vi "Final.vi"(0 "laser1":i32, 1 "laser2":i32, 2 "User1_float":dbl, 3 "Mode":i32, 4 "laser3":i32, 5 "laser4":i32, 6 "User2_int":i32, 7 "k":i32=1, 8 "If Scanning":dbl format="%#_13g", 9 "DC Offset X":dbl=5.0 format="%#_13g", 10 "ExposureTime(ms)":dbl, 12 "TriggerDelay(ms)":dbl=100.0, 13 "LoopDelay(second)":dbl, 14 "DC Offset Y":dbl=5.0 format="%#_13g", 15 "VoltageScanningChannel":tag="Dev2/ao0:3", 16 "LaserTriggerChannel":tag="Dev2/port0", 17 "frequency":dbl=30.0 caption="Frequency" format="%.6f", 18 "VXPX":dbl=0.08805 format="%#_13g", 19 "VYPY":dbl=0.10448 format="%#_13g", 20 "z_num":dbl format="%#_13g", 21 "delta_z(x1um)":dbl format="%#_13g", 22 "XShiftRatio":dbl=-0.01 format="%#_13g", 23 "YShiftRatio":dbl=0.01258 format="%#_13g", 24 "停止":bool, 25 "RotationAlpha":dbl=23.3, 27 "RotationBeta":dbl=113.3) -> ()   [LabVIEW 2019]
uses:
  <vilib>/DAQmx/write.llb/DAQmx Write (Digital 1D U32 1Chan NSamp).vi
  <vilib>/DAQmx/write.llb/DAQmx Write (Analog 2D DBL NChan NSamp).vi
  <vilib>/DAQmx/create/channels.llb/DAQmx Create Channel (AO-Voltage-Basic).vi
  <vilib>/DAQmx/create/channels.llb/DAQmx Create Channel (DO-Digital Output).vi
  <vilib>/DAQmx/configure/timing.llb/DAQmx Timing (Sample Clock).vi
  <vilib>/DAQmx/miscellaneous.llb/DAQmx Fill In Error Info.vi
  <vilib>/DAQmx/create/channels.llb/DAQmx Create Channel (CO-Pulse Generation-Frequency).vi
  <vilib>/DAQmx/configure/timing.llb/DAQmx Timing (Implicit).vi
  Global 6.vi
panel:
  out "Laser_status":i32[](array[numeric])
  out "Camera_trigger":i32[](array[numeric])
  out "XY Graph":cluster{"Y":dbl[], "Y":dbl[]}[](graph) caption="XY图"
  out "Scanning_index":dbl[][](array[numeric])=[[0.005349794238683128, 0.005349794238683128, 0.005349794238683128, 0.005349794238683128, -0.0, -0.0, -0.0, -0.0, -0.005349794238683128, -0.005349794238683128, -0.005349794238683128, -0.005349794238683128, -0.005349794238683128, -0.005349794238683128, -0.005349794238683128, -0.005349794238683128, -0.005349794238683128, -0.005349794238683128, -0.005349794238683128, -0.005349794238683128, -0.0, -0.0, -0.0, -0.0, 0.005349794238683128, 0.005349794238683128, 0.005349794238683128, 0.005349794238683128, 0.005349794238683128, 0.005349794238683128, 0.005349794238683128, 0.005349794238683128, -0.0, -0.0, -0.0, -0.0], [0.0020833333333333333, 0.0020833333333333333, 0.0020833333333333333, 0.0020833333333333333, 0.0020833333333333333, 0.0020833333333333333, 0.0020833333333333333, 0.0020833333333333333, 0.0020833333333333333, 0.0020833333333333333, 0.0020833333333333333, 0.0020833333333333333, -0.0, -0.0, -0.0, -0.0, -0.0020833333333333333, -0.0020833333333333333, -0.0020833333333333333, -0.0020833333333333333, -0.0020833333333333333, -0.0020833333333333333, -0.0020833333333333333, -0.0020833333333333333, -0.0020833333333333333, -0.0020833333333333333, -0.0020833333333333333, -0.0020833333333333333, -0.0, -0.0, -0.0, -0.0, -0.0, -0.0, -0.0, -0.0]]
  out "Scanning_voltage":dbl[][](array[numeric])=[[0.005349794238683128, 0.005349794238683128, 0.005349794238683128, 0.005349794238683128, -0.0, -0.0, -0.0, -0.0, -0.005349794238683128, -0.005349794238683128, -0.005349794238683128, -0.005349794238683128, -0.005349794238683128, -0.005349794238683128, -0.005349794238683128, -0.005349794238683128, -0.005349794238683128, -0.005349794238683128, -0.005349794238683128, -0.005349794238683128, -0.0, -0.0, -0.0, -0.0, 0.005349794238683128, 0.005349794238683128, 0.005349794238683128, 0.005349794238683128, 0.005349794238683128, 0.005349794238683128, 0.005349794238683128, 0.005349794238683128, -0.0, -0.0, -0.0, -0.0], [0.0020833333333333333, 0.0020833333333333333, 0.0020833333333333333, 0.0020833333333333333, 0.0020833333333333333, 0.0020833333333333333, 0.0020833333333333333, 0.0020833333333333333, 0.0020833333333333333, 0.0020833333333333333, 0.0020833333333333333, 0.0020833333333333333, -0.0, -0.0, -0.0, -0.0, -0.0020833333333333333, -0.0020833333333333333, -0.0020833333333333333, -0.0020833333333333333, -0.0020833333333333333, -0.0020833333333333333, -0.0020833333333333333, -0.0020833333333333333, -0.0020833333333333333, -0.0020833333333333333, -0.0020833333333333333, -0.0020833333333333333, -0.0, -0.0, -0.0, -0.0, -0.0, -0.0, -0.0, -0.0]]
  out "z_voltage":dbl[](array[numeric])
  out "Scanning_voltage_correct":dbl[][](array[numeric])=[[0.005349794238683128, 0.005349794238683128, 0.005349794238683128, 0.005349794238683128, -0.0, -0.0, -0.0, -0.0, -0.005349794238683128, -0.005349794238683128, -0.005349794238683128, -0.005349794238683128, -0.005349794238683128, -0.005349794238683128, -0.005349794238683128, -0.005349794238683128, -0.005349794238683128, -0.005349794238683128, -0.005349794238683128, -0.005349794238683128, -0.0, -0.0, -0.0, -0.0, 0.005349794238683128, 0.005349794238683128, 0.005349794238683128, 0.005349794238683128, 0.005349794238683128, 0.005349794238683128, 0.005349794238683128, 0.005349794238683128, -0.0, -0.0, -0.0, -0.0], [0.0020833333333333333, 0.0020833333333333333, 0.0020833333333333333, 0.0020833333333333333, 0.0020833333333333333, 0.0020833333333333333, 0.0020833333333333333, 0.0020833333333333333, 0.0020833333333333333, 0.0020833333333333333, 0.0020833333333333333, 0.0020833333333333333, -0.0, -0.0, -0.0, -0.0, -0.0020833333333333333, -0.0020833333333333333, -0.0020833333333333333, -0.0020833333333333333, -0.0020833333333333333, -0.0020833333333333333, -0.0020833333333333333, -0.0020833333333333333, -0.0020833333333333333, -0.0020833333333333333, -0.0020833333333333333, -0.0020833333333333333, -0.0, -0.0, -0.0, -0.0, -0.0, -0.0, -0.0, -0.0]]
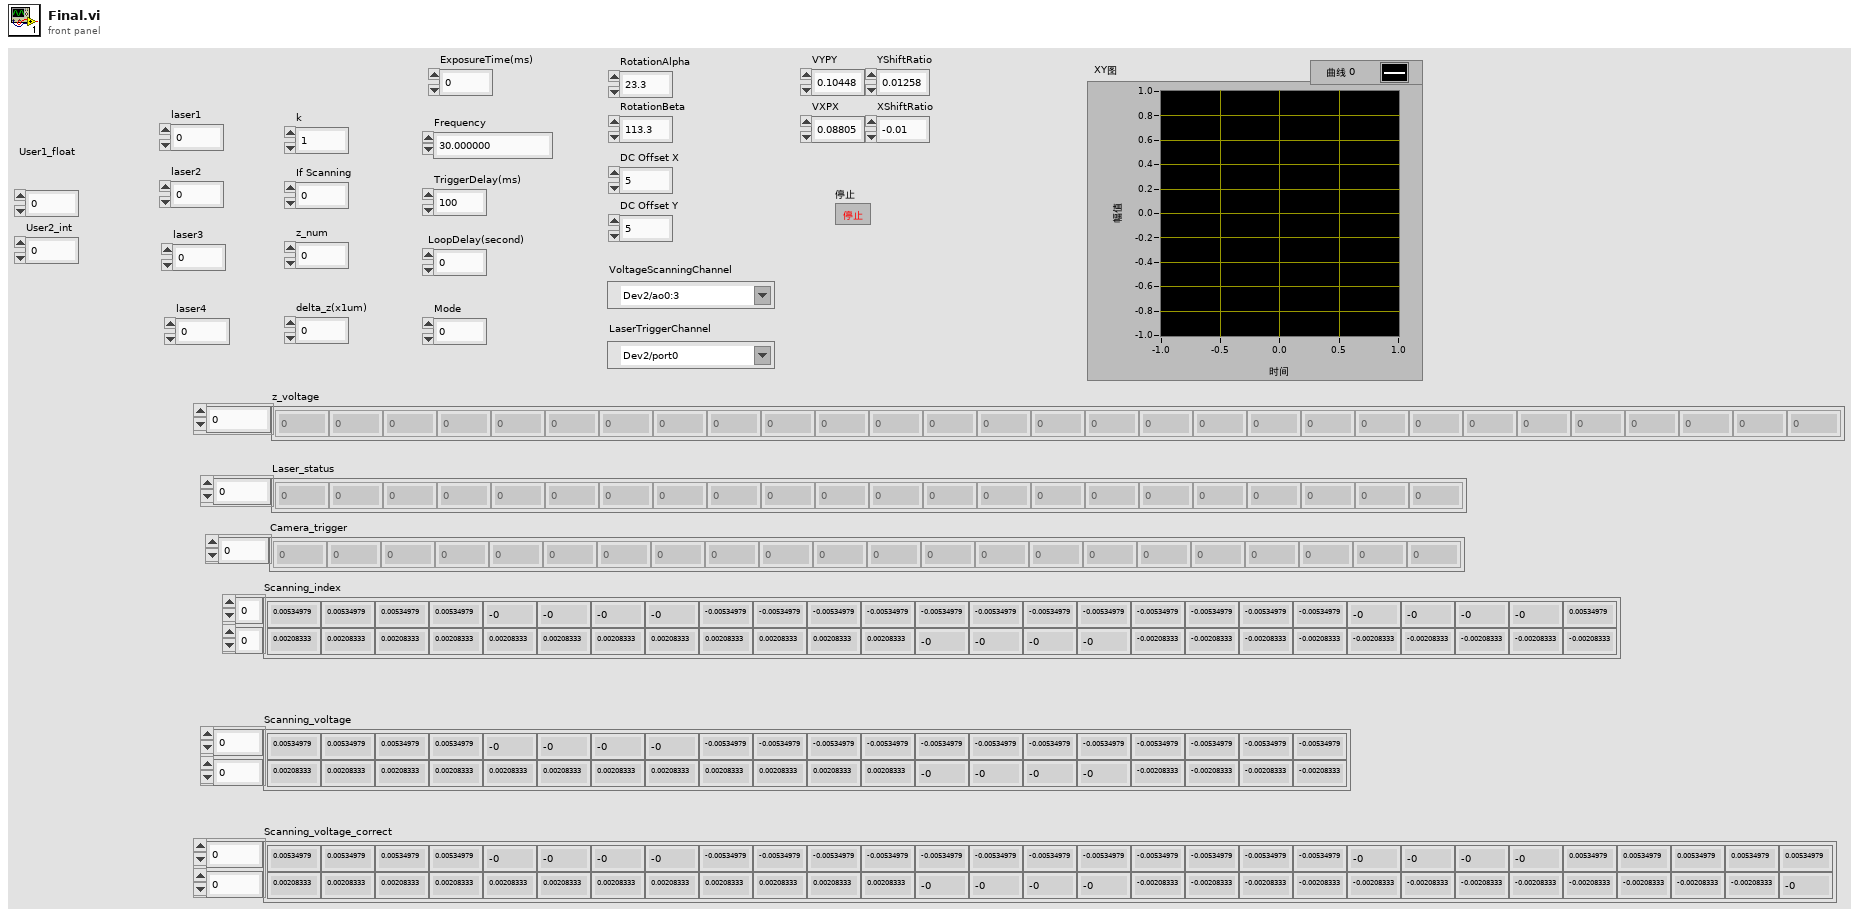
[diagram p1: front panel]
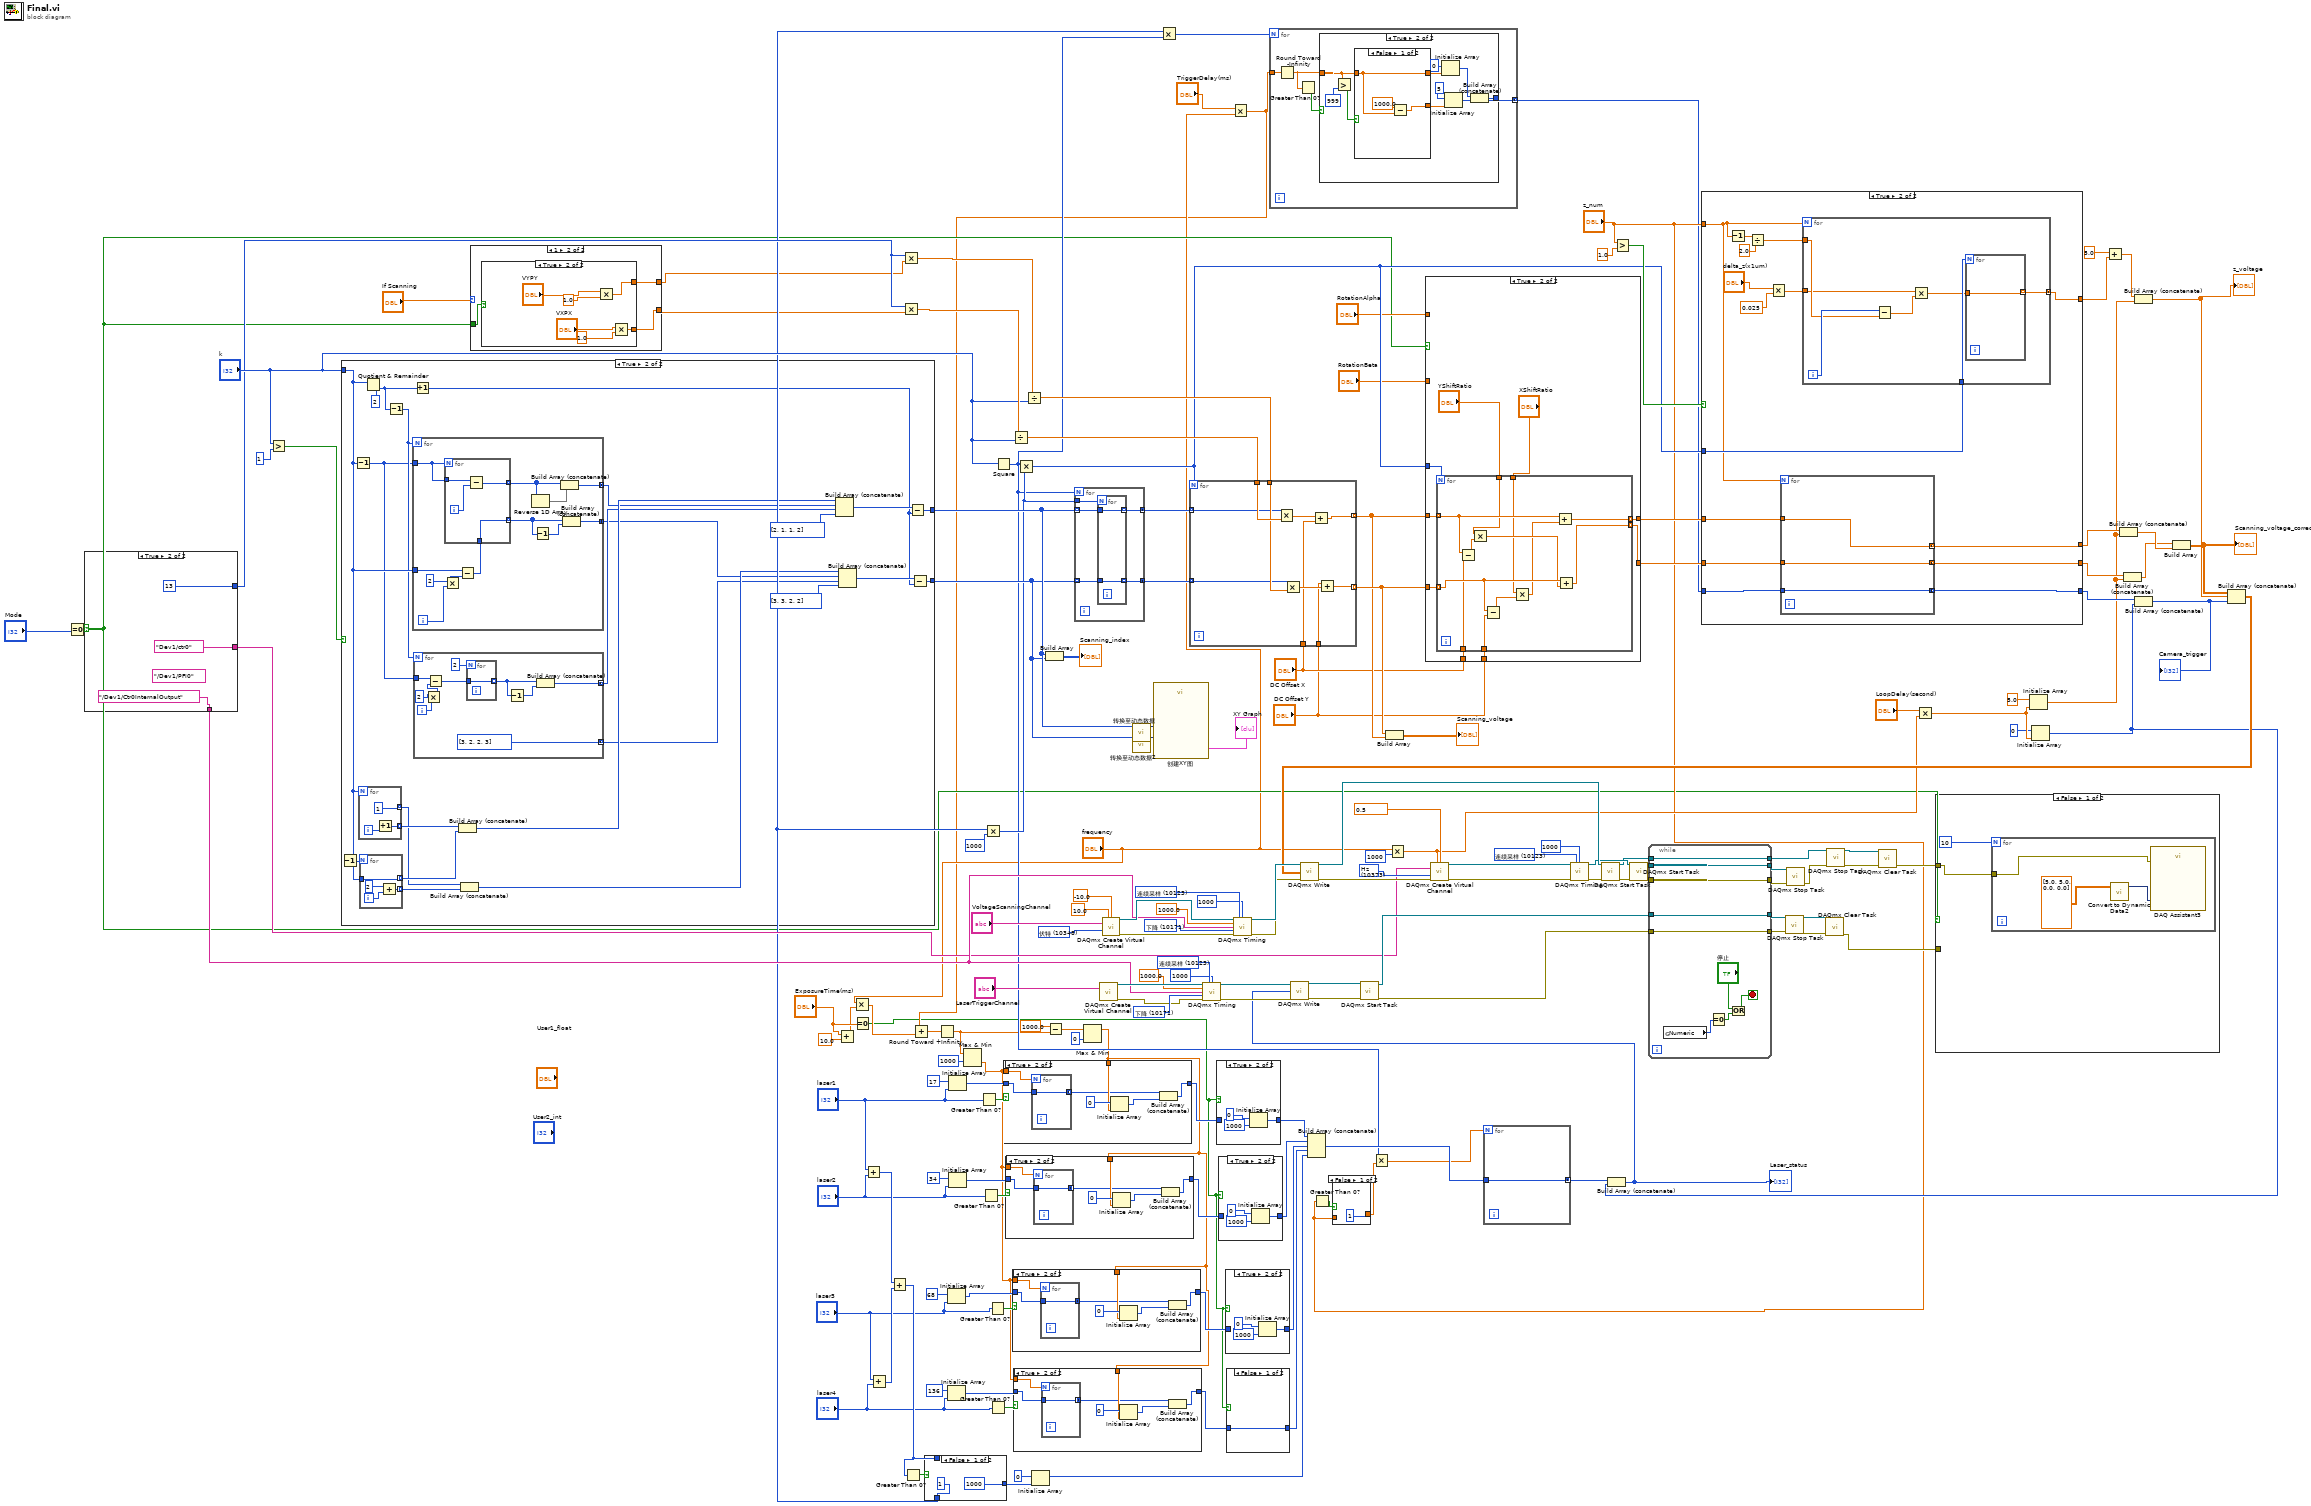
[diagram p0: block diagram]
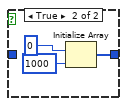
[diagram p2: hidden frame]
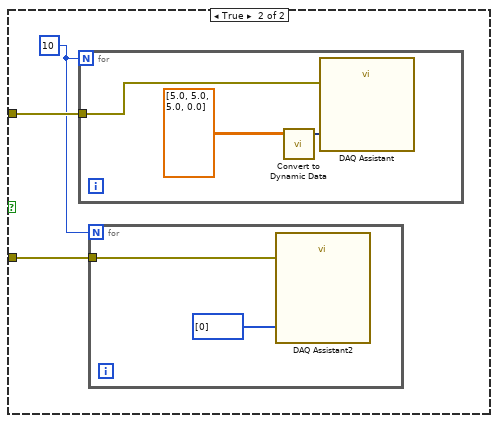
[diagram p10: hidden frame]
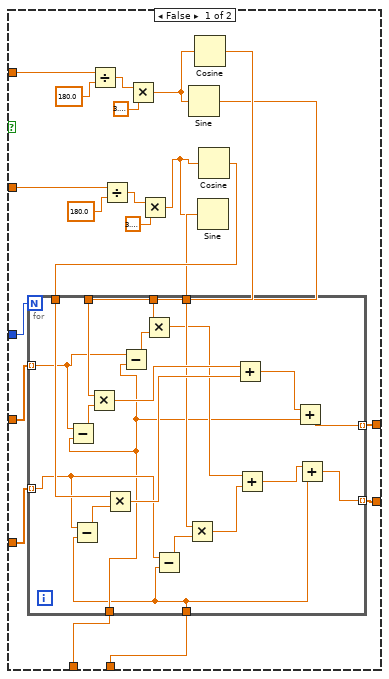
[diagram p11: hidden frame]
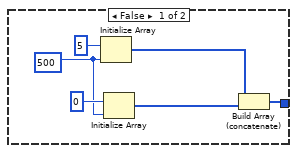
[diagram p12: hidden frame]
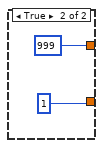
[diagram p13: hidden frame]
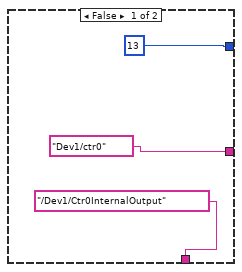
[diagram p14: hidden frame]
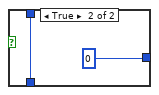
[diagram p16: hidden frame]
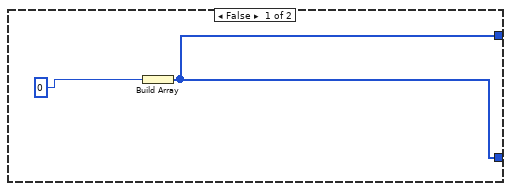
[diagram p17: hidden frame]
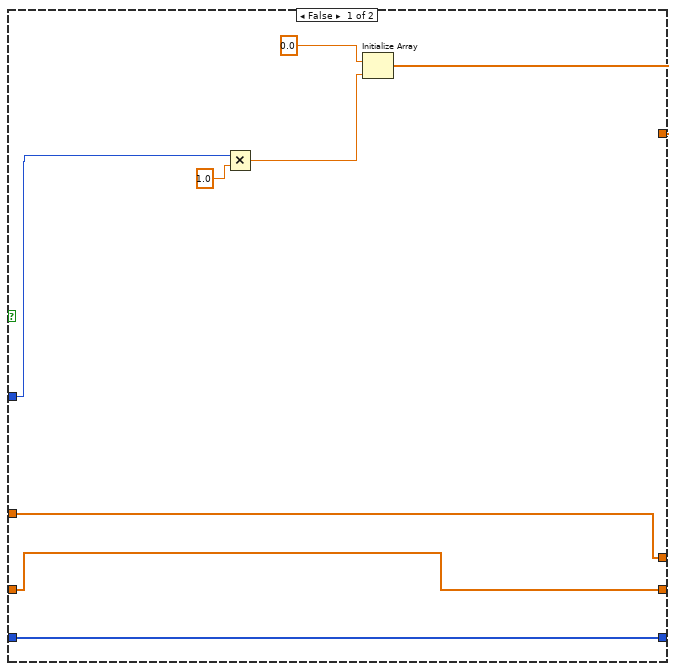
[diagram p18: hidden frame]
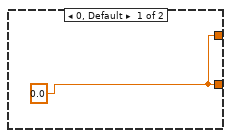
[diagram p19: hidden frame]
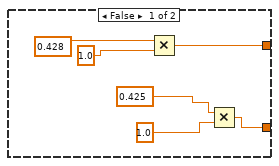
[diagram p20: hidden frame]
diagram:
  w134 = 10171 items=["上升"=10280, "下降"=10171] ("active edge")
  w136 = 10123 items=["有限采样"=10178, "连续采样"=10123, "硬件定时单点"=12522] ("sample mode")
  w148 = 10123 items=["有限采样"=10178, "连续采样"=10123, "硬件定时单点"=12522] ("sample mode")
  w159 = 10373 items=["Hz"=10373] ("units")
  w161 = 10348 items=["伏特"=10348, "来自自定义换算"=10065] ("units")
  w164 = 10171 items=["上升"=10280, "下降"=10171] ("active edge")
  w166 = 10123 items=["有限采样"=10178, "连续采样"=10123, "硬件定时单点"=12522] ("sample mode")
  n1 = Equal To 0?(x="Mode") -> (x = 0?=w40:bool)
  n2 = case shown="True" w40 {
    tunnel: [13 13] -> w55
    tunnel: [tag "/Dev1/Ctr0InternalOutput" ("source") tag "/Dev1/Ctr0InternalOutput" ("source")] -> w54
    tunnel: [tag "Dev1/ctr0" ("counter") tag "Dev1/ctr0" ("counter")] -> w52
    frame False {
    }
    frame True {
      (unwired) tag "/Dev1/PFI0" ("source")
    }
  }
  n3 = Greater?(x="k", y=1) -> (0:w95:bool)
  n4 = case shown="True" w95 {
    tunnel: "k" -> [_ w191]
    tunnel: [w173 w176] -> w101
    tunnel: [w173 w175] -> w99
    frame False {
      n5 = Build Array(0) -> (w173:i32[])
    }
    frame True {
      n6 = Decrement(x=w191) -> (x-1=w196:i32)
      n7 = Decrement(x=w191) -> (x-1=w189:i32)
      n8 = for {
        N: w191 -> [_]
        tunnel: [1] -> w193 mode=indexing
        tunnel: [w229] -> w195 mode=indexing
        i -> [w230]
        n9 = Increment(x=w230) -> (x+1=w229:i32)
      }
      n10 = for {
        N: w196 -> [_]
        tunnel: [w228] -> w194 mode=indexing
        tunnel: w191 -> [w228]
        tunnel: [w225] -> w192 mode=indexing
        i -> [w227]
        n11 = Add(x=2, y=w227) -> (x+y=w225:i32)
      }
      n12 = Quotient & Remainder(x=w191, y=2) -> (floor(x/y)=w180:i32)  [unwired: 1 out]
      n13 = Decrement(x=w180) -> (x-1=w190:i32)
      n14 = for {
        N: w190 -> [_]
        tunnel: w189 -> [w220]
        tunnel: [w217] -> w187 mode=concatenating
        tunnel: w191 -> [w215]
        tunnel: [w209] -> w182 mode=concatenating
        i -> [w213]
        n15 = Multiply(x=2, y=w213) -> (x*y=w216:i32)
        n16 = Subtract(x=w215, y=w216) -> (x-y=w212:i32)
        n17 = for {
          N: w220 -> [_]
          tunnel: w220 -> [w224]
          tunnel: [w223] -> w218 mode=indexing
          tunnel: w212 -> [w221]
          tunnel: [w221] -> w211 mode=indexing
          i -> [w222]
          n18 = Subtract(x=w224, y=w222) -> (x-y=w223:i32)
        }
        n19 = Reverse 1D Array(array=w218) -> (reversed array=w219:i32[])
        n20 = Decrement(x=w211) -> (x-1=w210:i32[])
        n21 = Build Array (concatenate)(w218, w219) -> (w217:i32[])
        n22 = Build Array (concatenate)(w211, w210) -> (w209:i32[])
      }
      n23 = Increment(x=w180) -> (x+1=w177:i32)
      n24 = for {
        N: w190 -> [_]
        tunnel: w189 -> [w206]
        tunnel: [w202] -> w186 mode=concatenating
        tunnel: [i32[] [3, 2, 2, 3]] -> w181 mode=concatenating
        i -> [w200]
        n25 = Multiply(x=2, y=w200) -> (x*y=w198:i32)
        n26 = Subtract(x=w206, y=w198) -> (x-y=w205:i32)
        n27 = for {
          N: 2 -> [_]
          tunnel: [w208] -> w203 mode=indexing
          tunnel: w205 -> [w208]
        }
        n28 = Decrement(x=w203) -> (x-1=w204:i32[])
        n29 = Build Array (concatenate)(w203, w204) -> (w202:i32[])
      }
      n30 = Build Array (concatenate)(w195, w194) -> (w188:i32[])
      n31 = Build Array (concatenate)(w193, w192) -> (w183:i32[])
      n32 = Build Array (concatenate)(w188, w187, w186, i32[] [2, 1, 1, 2]) -> (w179:i32[])
      n33 = Build Array (concatenate)(w183, w182, w181, i32[] [3, 3, 2, 2]) -> (w178:i32[])
      n34 = Subtract(x=w179, y=w177) -> (x-y=w176:i32[])
      n35 = Subtract(x=w178, y=w177) -> (x-y=w175:i32[])
    }
  }
  n36 = case shown="1" "If Scanning" {
    tunnel: [w232 w234] -> w44
    tunnel: [w232 w235] -> w43
    tunnel: w40 -> [_ w233]
    frame 0, Default {
      w232 = 0.0
    }
    frame 1 {
      n37 = case shown="True" w233 {
        tunnel: [w236 w246] -> w235
        tunnel: [w237 w244] -> w234
        frame False {
          n38 = Multiply(x=0.428, y=1.0 ("ratio_y")) -> (x*y=w237:dbl)
          n39 = Multiply(x=0.425 ("y"), y=1.0 ("ratio_x")) -> (x*y=w236:dbl)
        }
        frame True {
          n40 = Multiply(x="VYPY", y=1.0) -> (x*y=w244:dbl)
          n41 = Multiply(x="VXPX", y=1.0) -> (x*y=w246:dbl)
        }
      }
    }
  }
  n42 = Add(x="ExposureTime(ms)", y=10.0) -> (x+y=w1:dbl)
  n43 = Multiply(x="frequency", y=w1) -> (x*y=w35:dbl)
  n44 = Equal To 0?(x="ExposureTime(ms)") -> (x = 0?=w12:bool)
  n45 = Add(x="laser1", y="laser2") -> (x+y=w86:i32)
  n46 = Add(x="laser3", y="laser4") -> (x+y=w85:i32)
  n47 = Add(x=w86, y=w85) -> (x+y=w81:i32)
  n48 = Multiply(x=w55, y=w44) -> (x*y=w140:dbl)
  n49 = Multiply(x=w55, y=w43) -> (x*y=w142:dbl)
  n50 = Greater Than 0?(x=w81) -> (x > 0?=w82:bool)
  n51 = case shown="False" w82 {
    tunnel: [1000 0] -> w83
    tunnel: [1 w250] -> w49
    tunnel: w81 -> [_ w250]
    frame False {
    }
    frame True {
    }
  }
  n52 = Initialize Array(68, "laser3") -> (w18:i32[])
  n53 = Initialize Array(136, "laser4") -> (w17:i32[])
  n54 = Initialize Array(17, "laser1") -> (w37:i32[])
  n55 = Initialize Array(34, "laser2") -> (w24:i32[])
  n56 = Greater Than 0?(x="laser1") -> (x > 0?=w38:bool)
  n57 = Greater Than 0?(x="laser2") -> (x > 0?=w26:bool)
  n58 = Multiply(x=w49, y=1000) -> (x*y=w79:i32)
  n59 = Greater Than 0?(x="laser3") -> (x > 0?=w22:bool)
  n60 = Greater Than 0?(x="laser4") -> (x > 0?=w20:bool)
  n61 = Square(x="k") -> (x^2=w48:i32)
  n62 = Divide(x=w142, y="k") -> (x/y=w141:dbl)
  n63 = Multiply(x=w48, y=w79) -> (x*y=w78:i32)
  n64 = Divide(x=w140, y="k") -> (x/y=w139:dbl)
  n65 = Initialize Array(0, w83) -> (w53:i32[])
  n66 = Build Array(w101, w99) -> (→"Scanning_index":i32[][])
  n67 = for {
    N: w48 -> [_]
    tunnel: w101 -> [w255] mode=indexing
    tunnel: [w254] -> w105 mode=concatenating
    tunnel: [w253] -> w104 mode=concatenating
    tunnel: w99 -> [w252] mode=indexing
    tunnel: w79 -> [w256]
    n68 = for {
      N: w256 -> [_]
      tunnel: [w258] -> w254 mode=indexing
      tunnel: w255 -> [w258]
      tunnel: [w257] -> w253 mode=indexing
      tunnel: w252 -> [w257]
    }
  }
  n69 = call-poly <vilib>:"DAQmx Create Virtual Channel.vi"("lines"="LaserTriggerChannel") -> ("task out"=w137:refnum<k21>, "error out"=w133:errorcluster)  [unwired: 13 in]
  n70 = call-poly <vilib>:"DAQmx Create Virtual Channel.vi"("maximum value"=10.0, "minimum value"=-10.0, "physical channels"="VoltageScanningChannel", "units"=w161) -> ("task out"=w138:refnum<k21>, "error out"=w160:errorcluster)  [unwired: 10 in]
  n71 = call "转换至动态数据"("Array"=w101) -> ("Dynamic Data Type"=w100:dynamicdata)  [unwired: 3 in]
  n72 = call "转换至动态数据2"("Array"=w99) -> ("Dynamic Data Type"=w98:dynamicdata)  [unwired: 3 in]
  n73 = call "创建XY图"("Y Input"=w98, "X Input"=w100) -> ("XY Graph"=→"XY Graph":cluster{"X":dbl[], "Y":dbl[]}[])  [unwired: 8 in, 1 out]
  n74 = Multiply(x=w49, y=w48) -> (x*y=w50:i32)
  n75 = for {
    N: w78 -> [_]
    tunnel: w105 -> [w260] mode=indexing
    tunnel: w104 -> [w259] mode=indexing
    tunnel: [w263] -> w111 mode=indexing
    tunnel: [w264] -> w112 mode=indexing
    tunnel: w139 -> [w267]
    tunnel: w141 -> [w268]
    tunnel: "DC Offset X" -> [w262]
    tunnel: "DC Offset Y" -> [w261]
    n76 = Multiply(x=w260, y=w268) -> (x*y=w266:dbl)
    n77 = Multiply(x=w259, y=w267) -> (x*y=w265:dbl)
    n78 = Add(x=w266, y=w262) -> (x+y=w263:dbl)
    n79 = Add(x=w261, y=w265) -> (x+y=w264:dbl)
  }
  n80 = call-poly <vilib>:"DAQmx Timing.vi"("task/channels in"=w137, "sample mode"=w136, "samples per channel"=1000, "rate"=1000.0, "source"=w54, "active edge"=w134, "error in"=w133) -> ("task out"=w132:refnum<k21>, "error out"=w131:errorcluster)  [unwired: 7 in]
  n81 = Multiply(x="TriggerDelay(ms)", y="frequency") -> (x*y=w34:dbl)
  n82 = Add(x=w34, y=w35) -> (x+y=w4:dbl)
  n83 = Round Toward +Infinity(x=w4) -> (ceil(x): smallest int >= x=w29:dbl)
  n84 = Max & Min(x=w29, y=1000) -> (min(x,y)=w14:dbl)  [unwired: 1 out]
  n85 = Subtract(x=1000.0, y=w29) -> (x-y=w31:dbl)
  n86 = Max & Min(x=w31, y=0) -> (max(x,y)=w13:dbl)  [unwired: 1 out]
  n87 = case shown="True" w38 {
    tunnel: [w269 w270] -> w27
    tunnel: w37 -> [w269 w276]
    tunnel: w14 -> [_ w275]
    tunnel: w13 -> [_ w273]
    frame False {
    }
    frame True {
      n88 = for {
        N: w275 -> [_]
        tunnel: [w277] -> w272 mode=concatenating
        tunnel: w276 -> [w277]
      }
      n89 = Initialize Array(0 ("element"), w273) -> (w271:i32[])
      n90 = Build Array (concatenate)(w272, w271) -> (w270:i32[])
    }
  }
  n91 = case shown="True" w26 {
    tunnel: [w278 w279] -> w25
    tunnel: w24 -> [w278 w285]
    tunnel: w14 -> [_ w284]
    tunnel: w13 -> [_ w282]
    frame False {
    }
    frame True {
      n92 = for {
        N: w284 -> [_]
        tunnel: [w286] -> w281 mode=concatenating
        tunnel: w285 -> [w286]
      }
      n93 = Initialize Array(0 ("element"), w282) -> (w280:i32[])
      n94 = Build Array (concatenate)(w281, w280) -> (w279:i32[])
    }
  }
  n95 = case shown="True" w22 {
    tunnel: [w287 w288] -> w21
    tunnel: w18 -> [w287 w294]
    tunnel: w14 -> [_ w293]
    tunnel: w13 -> [_ w291]
    frame False {
    }
    frame True {
      n96 = for {
        N: w293 -> [_]
        tunnel: [w295] -> w290 mode=concatenating
        tunnel: w294 -> [w295]
      }
      n97 = Initialize Array(0 ("element"), w291) -> (w289:i32[])
      n98 = Build Array (concatenate)(w290, w289) -> (w288:i32[])
    }
  }
  n99 = case shown="True" w20 {
    tunnel: [w296 w297] -> w19
    tunnel: w17 -> [w296 w303]
    tunnel: w14 -> [_ w302]
    tunnel: w13 -> [_ w300]
    frame False {
    }
    frame True {
      n100 = for {
        N: w302 -> [_]
        tunnel: [w304] -> w299 mode=concatenating
        tunnel: w303 -> [w304]
      }
      n101 = Initialize Array(0 ("element"), w300) -> (w298:i32[])
      n102 = Build Array (concatenate)(w299, w298) -> (w297:i32[])
    }
  }
  n103 = case shown="True" w12 {
    tunnel: [w305 w306] -> w28
    tunnel: w27 -> [w305 _]
    frame False {
    }
    frame True {
      n104 = Initialize Array(0 ("element"), 1000 ("dimension size")) -> (w306:i32[])
    }
  }
  n105 = case shown="True" w12 {
    tunnel: [w309 w310] -> w11
    tunnel: w25 -> [w309 _]
    frame False {
    }
    frame True {
      n106 = Initialize Array(0 ("element"), 1000 ("dimension size")) -> (w310:i32[])
    }
  }
  n107 = case shown="True" w12 {
    tunnel: [w313 w314] -> w10
    tunnel: w21 -> [w313 _]
    frame False {
    }
    frame True {
      n108 = Initialize Array(0 ("element"), 1000 ("dimension size")) -> (w314:i32[])
    }
  }
  n109 = case shown="False" w12 {
    tunnel: [w317 w318] -> w9
    tunnel: w19 -> [w317 _]
    frame False {
    }
    frame True {
      n110 = Initialize Array(0 ("element"), 1000 ("dimension size")) -> (w318:i32[])
    }
  }
  n111 = call-poly <vilib>:"DAQmx Timing.vi"("task/channels in"=w138, "sample mode"=w166, "samples per channel"=1000, "rate"=1000.0, "source"=w54, "active edge"=w164, "error in"=w160) -> ("task out"=w156:refnum<k21>, "error out"=w154:errorcluster)  [unwired: 7 in]
  n112 = for {
    N: w50 -> [_]
    tunnel: [w324] -> w47 mode=concatenating
    tunnel: w34 -> [w322]
    n113 = Round Toward -Infinity(1:w322) -> (0:w321:dbl)
    n114 = Greater Than 0?(x=w321) -> (x > 0?=w323:bool)
    n115 = case shown="True" w323 {
      tunnel: w321 -> [_ w333]
      tunnel: [w325 w336] -> w324
      frame False {
        w326 = 500
        n116 = Initialize Array(5, w326) -> (w328:i32[])
        n117 = Initialize Array(0, w326) -> (w327:i32[])
        n118 = Build Array (concatenate)(w328, w327) -> (w325:i32[])
      }
      frame True {
        n119 = Greater?(x=w333, y=999) -> (0:w335:bool)
        n120 = case shown="False" w335 {
          tunnel: w333 -> [w341 _]
          tunnel: [w342 1] -> w332
          tunnel: [w341 999] -> w331
          frame False {
            n121 = Subtract(x=1000.0, y=w341) -> (x-y=w342:dbl)
          }
          frame True {
          }
        }
        n122 = Initialize Array(0, w331) -> (w338:i32[])
        n123 = Initialize Array(5, w332) -> (w337:i32[])
        n124 = Build Array (concatenate)(w338, w337) -> (w336:i32[])
      }
    }
  }
  n125 = Build Array (concatenate)(w28, w11, w10, w9, w53) -> (w63:i32[])
  n126 = Greater Than 0?(x="z_num") -> (x > 0?=w60:bool)
  n127 = case shown="False" w60 {
    tunnel: "z_num" -> [_ w347]
    tunnel: [1 w347] -> w58
    frame False {
    }
    frame True {
    }
  }
  n128 = Multiply(x=w48, y=w58) -> (x*y=w57:dbl)
  n129 = Build Array(w112, w111) -> (→"Scanning_voltage":dbl[][])
  n130 = Multiply(x="frequency", y=1000) -> (x*y=w65:dbl)
  n131 = case shown="True" w40 {
    tunnel: w112 -> [w353 w397]
    tunnel: w111 -> [w354 w396]
    tunnel: [w348 w395] -> w109
    tunnel: [w352 w394] -> w108
    tunnel: w78 -> [w351 w393]
    tunnel: "DC Offset X" -> [w356 w392]
    tunnel: "DC Offset Y" -> [w355 w391]
    tunnel: "RotationAlpha" -> [w350 _]
    tunnel: "RotationBeta" -> [w349 _]
    frame False {
      n132 = Divide(x=w350, y=180.0) -> (x/y=w364:dbl)
      n133 = Divide(x=w349, y=180.0) -> (x/y=w360:dbl)
      n134 = Multiply(x=w364, y=3.141592653589793) -> (x*y=w361:dbl)
      n135 = Multiply(x=w360, y=3.141592653589793) -> (x*y=w357:dbl)
      n136 = Sine(x=w361) -> (sin(x)=w366:dbl)
      n137 = Cosine(x=w361) -> (cos(x)=w368:dbl)
      n138 = Sine(x=w357) -> (sin(x)=w365:dbl)
      n139 = Cosine(x=w357) -> (cos(x)=w367:dbl)
      n140 = for {
        N: w351 -> [_]
        tunnel: w353 -> [w377] mode=indexing
        tunnel: w354 -> [w380] mode=indexing
        tunnel: [w372] -> w348 mode=indexing
        tunnel: [w371] -> w352 mode=indexing
        tunnel: w368 -> [w385]
        tunnel: w367 -> [w384]
        tunnel: w366 -> [w379]
        tunnel: w365 -> [w378]
        tunnel: w356 -> [w373]
        tunnel: w355 -> [w369]
        n141 = Subtract(x=w380, y=w373) -> (x-y=w388:dbl)
        n142 = Subtract(x=w377, y=w369) -> (x-y=w387:dbl)
        n143 = Multiply(x=w385, y=w388) -> (x*y=w383:dbl)
        n144 = Multiply(x=w384, y=w387) -> (x*y=w386:dbl)
        n145 = Subtract(x=w380, y=w373) -> (x-y=w382:dbl)
        n146 = Multiply(x=w379, y=w382) -> (x*y=w375:dbl)
        n147 = Subtract(x=w377, y=w369) -> (x-y=w381:dbl)
        n148 = Multiply(x=w378, y=w381) -> (x*y=w376:dbl)
        n149 = Add(x=w383, y=w386) -> (x+y=w374:dbl)
        n150 = Add(x=w375, y=w376) -> (x+y=w370:dbl)
        n151 = Add(x=w374, y=w373) -> (x+y=w372:dbl)
        n152 = Add(x=w370, y=w369) -> (x+y=w371:dbl)
      }
    }
    frame True {
      n153 = for {
        N: w393 -> [_]
        tunnel: w397 -> [w406] mode=indexing
        tunnel: w396 -> [w408] mode=indexing
        tunnel: [w403] -> w395 mode=indexing
        tunnel: [w402] -> w394 mode=indexing
        tunnel: "YShiftRatio" -> [w401]
        tunnel: "XShiftRatio" -> [w400]
        tunnel: w392 -> [w399]
        tunnel: w391 -> [w398]
        n154 = Subtract(x=w408, y=w399) -> (x-y=w409:dbl)
        n155 = Multiply(x=w401, y=w409) -> (x*y=w405:dbl)
        n156 = Subtract(x=w406, y=w398) -> (x-y=w407:dbl)
        n157 = Multiply(x=w400, y=w407) -> (x*y=w404:dbl)
        n158 = Add(x=w408, y=w404) -> (x+y=w403:dbl)
        n159 = Add(x=w406, y=w405) -> (x+y=w402:dbl)
      }
    }
  }
  n160 = for {
    N: w57 -> [_]
    tunnel: w63 -> [w410]
    tunnel: [w410] -> w64 mode=concatenating
  }
  n161 = Greater?(x="z_num", y=1.0) -> (0:w106:bool)
  n162 = case shown="True" w106 {
    tunnel: w109 -> [w411 w427]
    tunnel: w108 -> [w412 w426]
    tunnel: w78 -> [w414 w425]
    tunnel: "z_num" -> [_ w424]
    tunnel: [w417 w423] -> w7
    tunnel: w47 -> [w413 w422]
    tunnel: [w413 w421] -> w68
    tunnel: [w411 w420] -> w72
    tunnel: [w412 w419] -> w71
    frame False {
      n163 = Multiply(x=w414, y=1.0) -> (x*y=w416:dbl)
      n164 = Initialize Array(0.0, w416) -> (w417:dbl[])
    }
    frame True {
      n165 = Decrement(x=w424) -> (x-1=w431:dbl)
      n166 = Divide(x=w431, y=2.0) -> (x/y=w429:dbl)
      n167 = Multiply(x="delta_z(x1um)", y=0.025) -> (x*y=w428:dbl)
      n168 = for {
        N: w424 -> [_]
        tunnel: w427 -> [w436]
        tunnel: w426 -> [w435]
        tunnel: [w436] -> w420 mode=concatenating
        tunnel: [w435] -> w419 mode=concatenating
        tunnel: w422 -> [w434]
        tunnel: [w434] -> w421 mode=concatenating
      }
      n169 = for {
        N: w424 -> [_]
        tunnel: w429 -> [w442]
        tunnel: w428 -> [w441]
        tunnel: w425 -> [w439]
        tunnel: [w437] -> w423 mode=concatenating
        i -> [w443]
        n170 = Subtract(x=w443, y=w442) -> (x-y=w440:dbl)
        n171 = Multiply(x=w441, y=w440) -> (x*y=w438:dbl)
        n172 = for {
          N: w439 -> [_]
          tunnel: [w444] -> w437 mode=indexing
          tunnel: w438 -> [w444]
        }
      }
    }
  }
  n173 = Multiply(x="LoopDelay(second)", y=w65) -> (x*y=w74:dbl)
  n174 = Initialize Array(5.0, w74) -> (w5:dbl[])
  n175 = Initialize Array(0, w74) -> (w62:i32[])
  n176 = Build Array (concatenate)(w64, w62) -> (w61:i32[])
  "Laser_status" <- w61
  n177 = call-poly <vilib>:"DAQmx Write.vi"("task/channels in"=w132, "data"=w61, "error in"=w131) -> ("task out"=w130:refnum<k21>, "error out"=w127:errorcluster)  [unwired: 10 in, 1 out]
  n178 = call <vilib>:"DAQmx Start Task.vi"("task/channels in"=w130, "error in"=w127) -> ("task out"=w129:refnum<k21>, "error out"=w124:errorcluster)  [unwired: 12 in]
  n179 = Add(x=5.0, y=w7) -> (x+y=w6:dbl[])
  n180 = Build Array (concatenate)(w72, w5) -> (w70:dbl[])
  n181 = Build Array (concatenate)(w71, w5) -> (w69:dbl[])
  n182 = Build Array (concatenate)(w6, w5) -> (w66:dbl[])
  "z_voltage" <- w66
  n183 = Build Array (concatenate)(w68, w62) -> (w67:i32[])
  "Camera_trigger" <- w67
  n184 = Build Array(w69, w70) -> (w77:dbl[][])
  "Scanning_voltage_correct" <- w77
  n185 = Build Array (concatenate)(w77, w66, w67) -> (w94:dbl[][])
  n186 = call-poly <vilib>:"DAQmx Write.vi"("task/channels in"=w156, "data"=w94, "error in"=w154) -> ("task out"=w155:refnum<k21>, "error out"=w153:errorcluster)  [unwired: 10 in, 1 out]
  n187 = call-poly <vilib>:"DAQmx Create Virtual Channel.vi"("frequency"=w65, "duty cycle"=0.5, "counter"=w52, "units"=w159, "error in"=w153) -> ("task out"=w150:refnum<k21>, "error out"=w144:errorcluster)  [unwired: 9 in]
  n188 = call-poly <vilib>:"DAQmx Timing.vi"("task/channels in"=w150, "sample mode"=w148, "samples per channel"=1000, "error in"=w144) -> ("task out"=w149:refnum<k21>, "error out"=w143:errorcluster)  [unwired: 10 in]
  n189 = call <vilib>:"DAQmx Start Task.vi"("task/channels in"=w155, "error in"=w143) -> ("task out"=w145:refnum<k21>, "error out"=w152:errorcluster)  [unwired: 12 in]
  n190 = call <vilib>:"DAQmx Start Task.vi"("task/channels in"=w149, "error in"=w152) -> ("task out"=w151:refnum<k21>, "error out"=w126:errorcluster)  [unwired: 12 in]
  n191 = while {
    tunnel: w151 -> [w453]
    tunnel: w126 -> [w450]
    tunnel: [w450] -> w119
    tunnel: [w453] -> w120
    tunnel: [w452] -> w146
    tunnel: w145 -> [w452]
    tunnel: w129 -> [w451]
    tunnel: [w451] -> w125
    tunnel: w124 -> [w449]
    tunnel: [w449] -> w123
    stop <- w446 stop-if-true
    n192 = global read "Global 6.vi" "Numeric"() -> (w445:i32)
    n193 = Equal To 0?(x=w445) -> (x = 0?=w448:bool)
    n194 = Or(x="停止", y=w448) -> (x .or. y?=w446:bool)
  }
  n195 = call <vilib>:"DAQmx Stop Task.vi"("task/channels in"=w125, "error in"=w123) -> ("task out"=w115:refnum<k21>, "error out"=w114:errorcluster)  [unwired: 12 in]
  n196 = call <vilib>:"DAQmx Stop Task.vi"("task/channels in"=w120, "error in"=w119) -> ("error out"=w118:errorcluster)  [unwired: 12 in, 1 out]
  n197 = call <vilib>:"DAQmx Clear Task.vi"("task in"=w115, "error in"=w114) -> ("error out"=w92:errorcluster)  [unwired: 13 in]
  n198 = call <vilib>:"DAQmx Stop Task.vi"("task/channels in"=w146, "error in"=w118) -> ("task out"=w117:refnum<k21>, "error out"=w116:errorcluster)  [unwired: 12 in]
  n199 = call <vilib>:"DAQmx Clear Task.vi"("task in"=w117, "error in"=w116) -> ("error out"=w93:errorcluster)  [unwired: 13 in]
  n200 = case shown="False" w40 {
    tunnel: w93 -> [w455 w461]
    tunnel: w92 -> [_ w460]
    frame False {
      n201 = for {
        N: 10 -> [_]
        tunnel: w455 -> [w456]
        n202 = call "Convert to Dynamic Data2"("2D Array"=dbl[][] [[5.0], [5.0], [0.0], [0.0]]) -> ("Dynamic Data Type"=w457:dynamicdata)  [unwired: 3 in]
        n203 = call "DAQ Assistant3"("data"=w457, "error in"=w456) -> ()  [unwired: 16 in, 2 out]
      }
    }
    frame True {
      w459 = 10
      n204 = for {
        N: w459 -> [_]
        tunnel: w461 -> [w466]
        n205 = call "Convert to Dynamic Data"("2D Array"=dbl[][] [[5.0], [5.0], [5.0], [0.0]]) -> ("Dynamic Data Type"=w464:dynamicdata)  [unwired: 3 in]
        n206 = call "DAQ Assistant"("data"=w464, "error in"=w466) -> ()  [unwired: 16 in, 2 out]
      }
      n207 = for {
        N: w459 -> [_]
        tunnel: w460 -> [w463]
        n208 = call "DAQ Assistant2"("data"=i32[] [0], "error in"=w463) -> ()  [unwired: 16 in, 2 out]
      }
    }
  }
